vi "SPI_TurnOffClockDivider.vi"(2 "error in (no error)":errorcluster, 3 "handle":u32) -> (0 "error out":errorcluster)   [LabVIEW 2013]
uses:
  lib/FTCSPI.dll
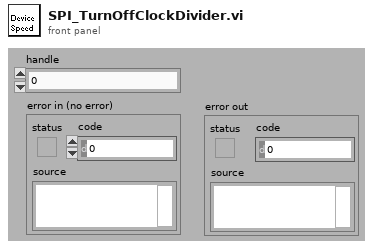
[diagram p1: front panel]
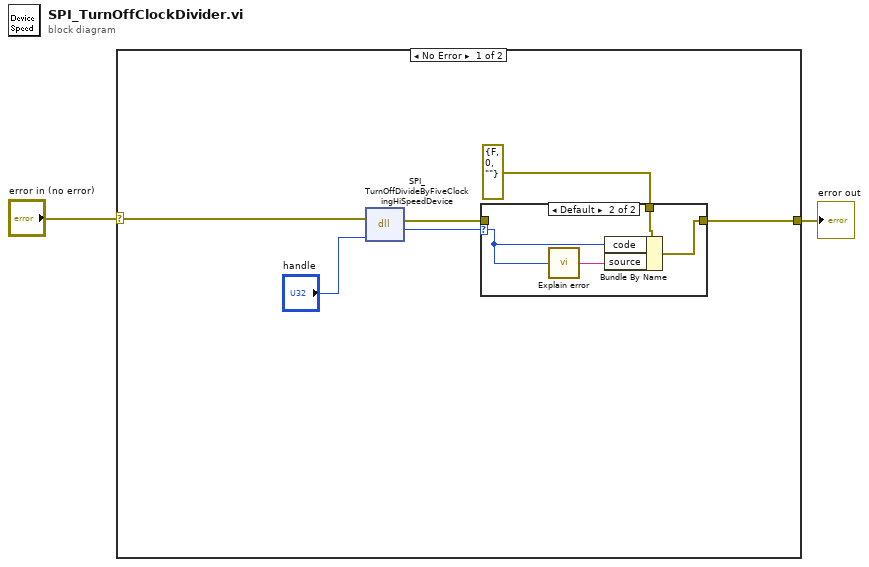
[diagram p0: block diagram]
diagram:
  n1 = case shown="No Error" "error in (no error)" {
    selector: "error in (no error)" -> [w5 w14]
    tunnel: [w4 w14] -> w1
    frame No Error {
      n2 = dll-call lib="C:/Users/SuperUser/Documents/HiSparc/hisparcdaq/FPGA/lib/FTCSPI.dll" fn="SPI_TurnOffDivideByFiveClockingHiSpeedDevice" label="SPI_SetHiSpeedDeviceGPIOs"(error in=w5, "handle"="handle") -> (error out=w6:errorcluster, "result"=w7:u32)  [unwired: 3 in, 1 out]
      n3 = case shown="Default" w7 {
        selector: w7 -> [_ w11]
        tunnel: w6 -> [w9 _]
        tunnel: [w9 w10] -> w4
        tunnel: errorcluster {"status"=FALSE, "code"=0, "source"=""} ("error out") -> [_ w13]
        frame 0 {
        }
        frame Default {
          n4 = call "Explain error.vi"("error"=w11) -> ("error string"=w12:string)
          n5 = Bundle By Name(cluster=w13, "code"=w11, "source"=w12) -> (w10:errorcluster)
        }
      }
    }
    frame Error {
    }
  }
  "error out" <- w1
